vi "FPGA_main_Ctrl_v1.vi"() -> ()   [LabVIEW 2020]
doc: "Main FPGA VI\n- AI, Signal conditioning\n- AO, Feedback linearization\n- Controller"
uses:
  Components/FPGA TypeDefs/SelectDirection_Enum.ctl
  Components/FPGA TypeDefs/SelectExcitation_Enum.ctl
  Components/FPGA TypeDefs/SelectAOchannel_Enum.ctl
  Components/Controller/TypeDefs/2ndOrderTFnum.ctl
  Components/Controller/TypeDefs/2ndOrderTFden.ctl
  <vilib>/rvi/Emulation/niFpgaGetClockAttributes.vi
  <vilib>/rvi/Emulation/niFpgaSctlEmulationGetInTimedLoop.vi
  <vilib>/rvi/Emulation/niFpgaEmulationReportErrorSimple.vi
  <vilib>/rvi/eio/common/nirviEmuTemplateMethod_errors.vi
  <vilib>/rvi/Emulation/niFpgaEmulationIsFPGAContextNoSignature.vi
  <vilib>/rvi/errors/niFpgaSetErrorForExecOnDevCompSimple.vi
  <vilib>/rvi/eio/common/nirviEmuReportErrorAndStop.vi
  <vilib>/rvi/DataTransferAndStorage/Container/Common/niFpgaContainerGetUniqueNameForEmu.vi
  <vilib>/rvi/FIFO/Fifo_Resource/nirvififoEmulationSetSize.vi
  <vilib>/rvi/FIFO/Fifo_Resource/nirviFifoEmulationQueueMgr.vi
  <instcachedir>/0/nirviFifoEmulationQueueMgr_E5CAEC123FF24DC58D834DCA3CDAA9B5.lvgen/nirviFifoEmulationQueueMgr_E5CAEC123FF24DC58D834DCA3CDAA9B5_001.vi
  <vilib>/rvi/FIFO/Fifo_Resource/nirvififoEmulationDetermineInputValidOut.vi
  <vilib>/rvi/FIFO/Fifo_Resource/nirvififoEmulationCreateLock.vi
  <vilib>/rvi/Emulation/niFpgaProcessEmulError.vi
  <vilib>/rvi/FIFO/Fifo_Resource/nirvififoEmulationObtainLock.vi
  <vilib>/rvi/FIFO/Fifo_Resource/nirvififoEmulationReleaseLock.vi
  <vilib>/rvi/occurrence/nirviWaitOnOccurrenceBase.vi
  <vilib>/rvi/errors/nirviReportUnexpectedCaseInternalError.vi
  <vilib>/rvi/errors/nirviReportUnexpectedCaseInternalError (U32).vi
  <vilib>/rvi/Emulation/niFpgaCriticalErrorInLSC.vi
  <vilib>/Utility/error.llb/Clear Errors.vi
  Components/PositionMeas/MovingAverage/256ptMovingAvg.vi
  Components/PositionMeas/MovingAverage/64ptMovingAvg.vi
  <vilib>/rvi/DataTransferAndStorage/Container/Common/niFpgaContainerSetEmuInfo.vi
  <vilib>/eio/EIONode/EIONode.xnode
  <vilib>/rvi/DataTransferAndStorage/Container/XNode/niFpgaContainer.xnode
  <vilib>/rvi/FIFO/Fifo_Resource/nirvififoEmulationWrite.vi
  <vilib>/rvi/FIFO/Fifo_Resource/nirvififoEmulationRead.vi
  <vilib>/rvi/FXPMathLib/FxpSub/XNode/nifxpmath_Sub.xnode
  <vilib>/rvi/FXPMathLib/FxpAdd/XNode/nifxpmath_Add.xnode
  <vilib>/rvi/LocalResourceManager/LocalResourceManager.xnode
  Components/PositionMeas/MovingAverage/MovingAvg.lvlib
  Components/PositionMeas/PositionMeas.lvlib
  Components/Controller/Controller.lvlib
  <vilib>/rvi/FXPMathLib/sim/FxpSim.dll
  Components/ReferenceGen/ReferenceGen.lvlib
  Components/CtrlEff/CtrlEff.lvlib
  Components/CtrlEff/Force2Volt/Force2Volt.lvlib
panel:
  in  "Numerator (b0, b1, b2) 5":T1=[0.0, 0.0, 0.0]
  in  "Denominator (a1, a2) 5":T2=[0.0, 0.0]
  in  "Denominator (a1, a2) 4":T2=[0.0, 0.0]
  in  "Denominator (a1, a2) 3":T2=[0.0, 0.0]
  in  "Denominator (a1, a2) 2":T2=[0.0, 0.0]
  in  "Numerator (b0, b1, b2) 4":T1=[0.0, 0.0, 0.0]
  in  "Numerator (b0, b1, b2) 3":T1=[0.0, 0.0, 0.0]
  in  "Numerator (b0, b1, b2) 2":T1=[0.0, 0.0, 0.0]
  in  "Denominator (a1, a2)":T2=[0.0, 0.0] format="%#_12g"
  in  "Numerator (b0, b1, b2)":T1=[0.0, 0.0, 0.0]
  in  "Current Sense Zero":fxp<+/-,25,5>[](array[numeric])=[0.0, 0.0, 0.0, 0.0, 0.0, 0.0]
  out "Total Ctrl Eff":fxp<+/-,25,5>[](array[numeric])
  in  "PosMeas_ZeroOffset":fxp<+/-,25,5>[](array[numeric])=[0.0, 0.0, 0.0, 0.0, 0.0]
  in  "AO enable?":bool
  out "Total PosRef":fxp<+/-,25,5>[](array[numeric])
  in  "Enable \nPos. Ref. Gen?":bool
  in  "Select Ref. direction":T3
  in  "PR Frequency [periods/tick]":fxp<+,32,0>
  in  "PR Amplitude [V]":fxp<+/-,25,5>
  in  "PR Excitation mode":T4
  out "Ref Gen Loop Time [ticks]":u32
  in  "Enable \nCtrl Eff dist?":bool
  in  "Enable \nAO dist?":bool
  in  "Select CE direction":T3
  in  "CE Frequency [periods/tick]":fxp<+,32,0>
  in  "CE Amplitude [V]":fxp<+/-,25,5>
  in  "CE Excitation mode":T4
  out "AO":fxp<+/-,20,5>[](array[numeric])
  in  "Run Controller?":bool
  in  "Ki*Ts":fxp<+,17,0>[](array[numeric])=[0.0, 0.0, 0.0, 0.0, 0.0] caption="Kp"
  out "U_Z,ThX,ThY,B,Bd":fxp<+/-,25,5>[](array[numeric])
  in  "Kp":fxp<+,17,17>[](array[numeric])=[0.0, 0.0, 0.0, 0.0, 0.0]
  out "Ctrl Loop\ntime [ticks]":u32
  in  "Z,ThX,ThY,B,Bd Ref":fxp<+/-,25,5>[](array[numeric])=[0.0, 0.0, 0.0, 0.0, 0.0]
  out "AI_HS":fxp<+/-,25,5>[](array[numeric])
  out "AI_LS":fxp<+/-,25,5>[](array[numeric])
  out "Z,ThX,ThY,B,Bd Meas":fxp<+/-,25,5>[](array[numeric])
  in  "Select AO channel":T5
  out "AO Loop time [ticks]":u32
  in  "AO Frequency [periods/tick]":fxp<+,32,0>
  in  "AO Amplitude [V]":fxp<+/-,25,5>
  in  "AO Excitation mode":T4
  out "AI LS 2 Loop time [ticks]":u32
  out "FPGA AI LS 2 FIFO\nOverflow?":bool
  out "AI LS 2 filter Loop time [ticks]":u32
  out "Current Sense":fxp<+/-,25,5>[](array[numeric])
  out "AI LS filter Loop time [ticks]":u32
  out "AI LS Loop time [ticks]":u16
  out "FPGA AI LS FIFO\nOverflow?":bool
  out "AI HS filter Loop time [ticks]":u32
  out "FPGA AI HS FIFO\nOverflow?":bool
  out "AI HS Loop time [ticks]":u32
  # "1 tick = 25 ns"
  # "2nd Order TF params"
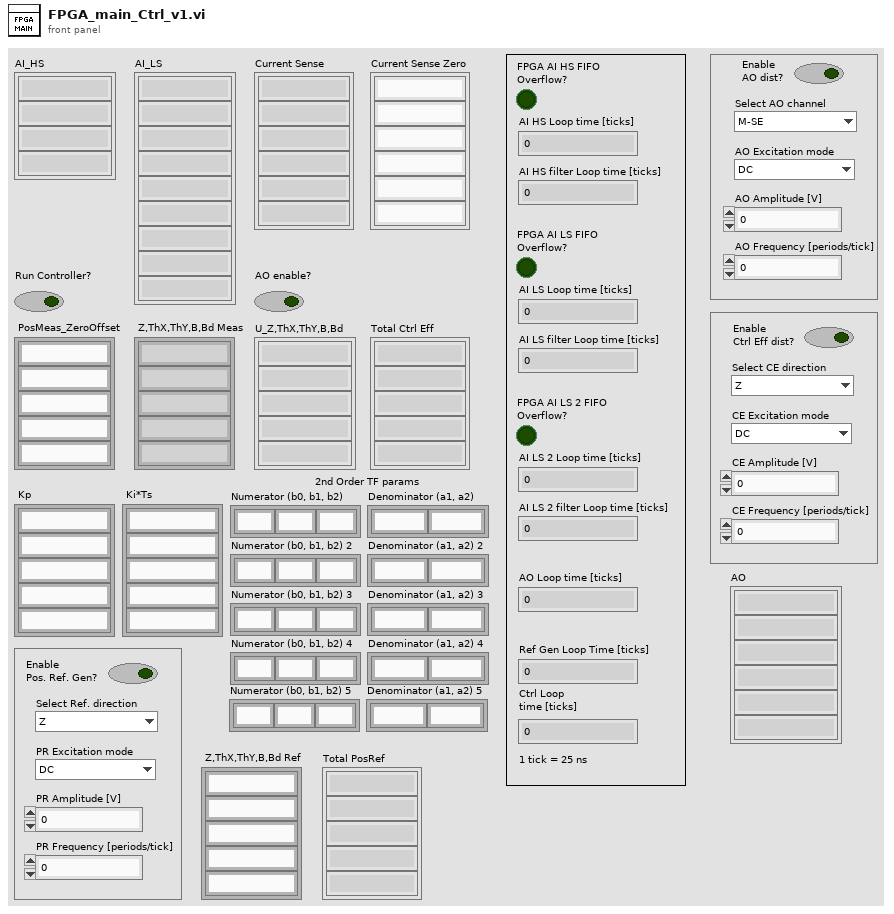
[diagram p1: front panel]
types:
  T1 = typedef "Controller.lvlib/2ndOrderTFnum.ctl" = fxp<+/-,28,2>[]
  T2 = typedef "Controller.lvlib/2ndOrderTFden.ctl" = fxp<+/-,28,2>[]
  T3 = typedef "SelectDirection_Enum.ctl" = enum8{"Z", "ThX", "ThY", "Bow", "B-d"}
  T4 = typedef "SelectExcitation_Enum.ctl" = enum8{"DC", "Sine", "Square", "WhiteNoise"}
  T5 = typedef "SelectAOchannel_Enum.ctl" = enum8{"M-SE", "M-NE", "M-NW", "M-SW", "M-CO", "M-CI"}
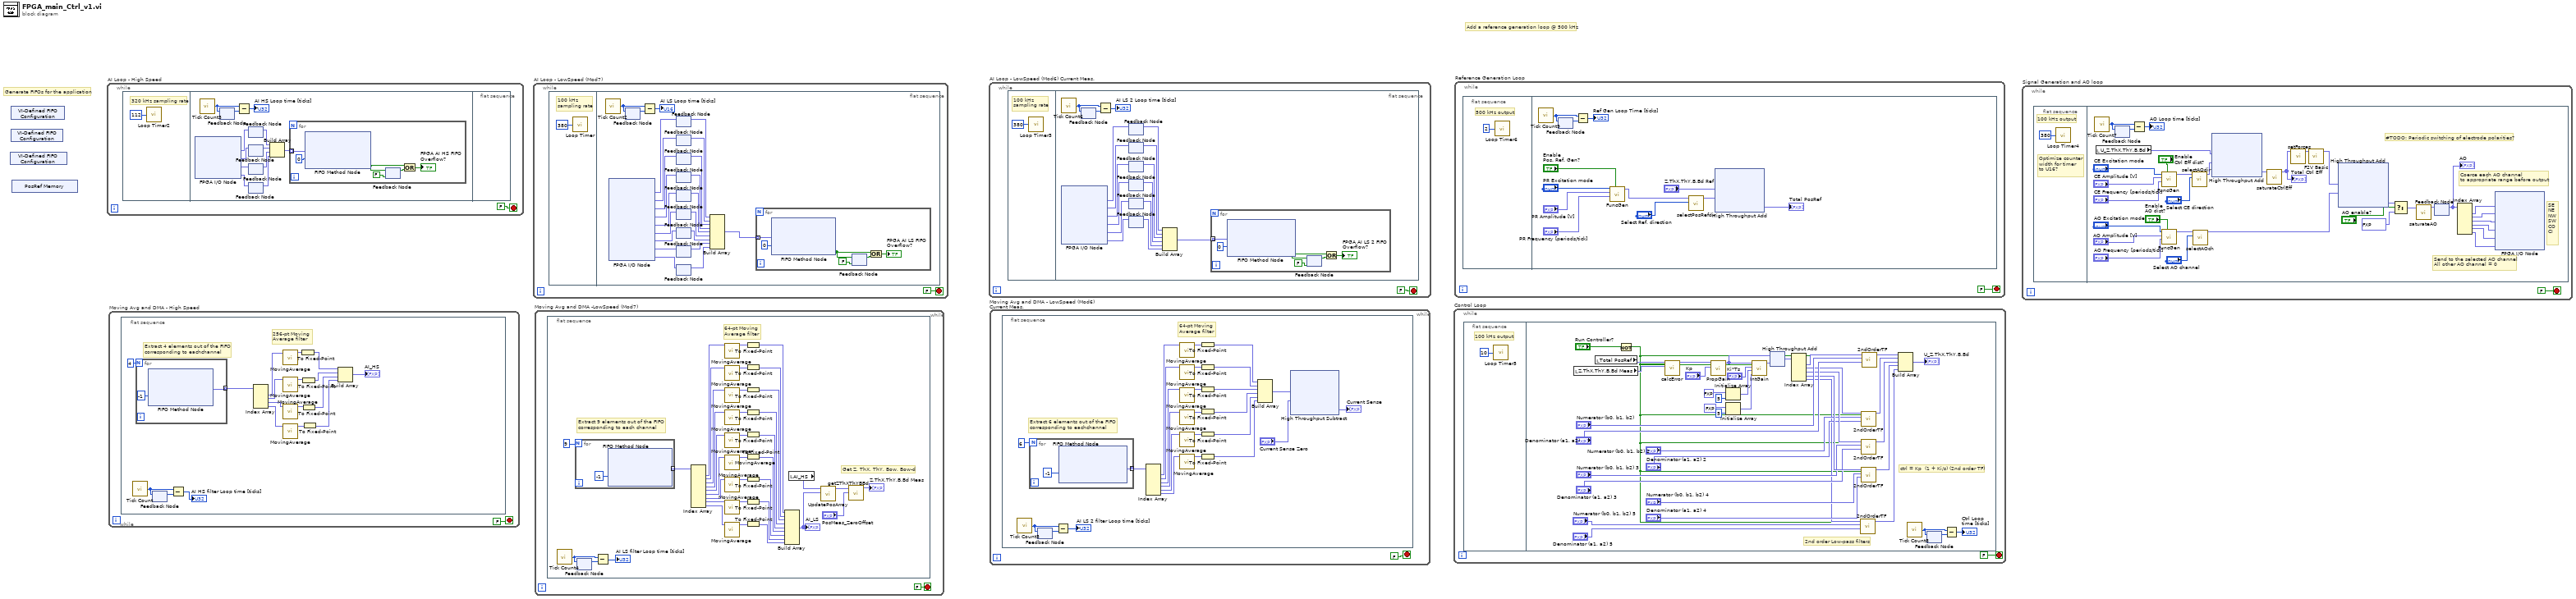
[diagram p0: block diagram]
diagram:
  # "Add a reference generation loop @ 500 kHz"
  # "Generate FIFOs for the application"
  n1 = xnode "VI-Defined FIFO Configuration"() -> ()  [unwired: 1 out]
  n2 = xnode "VI-Defined FIFO Configuration"() -> ()  [unwired: 1 out]
  n3 = xnode "VI-Defined FIFO Configuration"() -> ()  [unwired: 1 out]
  n4 = xnode "PosRef Memory"() -> ()  [unwired: 1 out]
  n5 = while "AI Loop - High Speed" {
    stop <- FALSE stop-if-true
    n6 = flat-sequence {
      frame #0 {
        # "320 kHz sampling rate"
        n7 = call "Loop Timer2"("Count(Ticks)"=u32 112) -> ()  [unwired: 1 out]
      }
      frame #1 {
        n8 = xnode "FPGA I/O Node"() -> ("Mod8/AI0"=w9:fxp<+/-,24,5>, "Mod8/AI1"=w8:fxp<+/-,24,5>, "Mod8/AI2"=w7:fxp<+/-,24,5>, "Mod8/AI3"=w6:fxp<+/-,24,5>)  [unwired: 4 in, 4 out]
        n9 = call "Tick Count3"() -> ("Tick Count(Ticks)"=w14:u32)
        n10 = feedback #1() -> (w13:u32)  [unwired: 1 in]
        n11 = feedback-in #1(w14) -> ()
        n12 = Subtract(x=w14, y=w13) -> (x-y=→"AI HS Loop time [ticks]":u32)
        n13 = feedback-in #2(w9) -> ()
        n14 = feedback #2() -> (w10:fxp<+/-,24,5>)  [unwired: 1 in]
        n15 = feedback #3() -> (w5:fxp<+/-,24,5>)  [unwired: 1 in]
        n16 = feedback-in #3(w8) -> ()
        n17 = feedback #4() -> (w4:fxp<+/-,24,5>)  [unwired: 1 in]
        n18 = feedback-in #4(w7) -> ()
        n19 = feedback #5() -> (w3:fxp<+/-,24,5>)  [unwired: 1 in]
        n20 = feedback-in #5(w6) -> ()
        n21 = Build Array(w10, w5, w4, w3) -> (w11:fxp<+/-,24,5>[])
        n22 = for {
          tunnel: w11 -> [w19] mode=indexing
          n23 = xnode ("FIFO Method Node")("Element"=w19, "Timeout"=0) -> ("Timed Out?"=w16:bool)  [unwired: 1 in, 1 out]
          n24 = feedback-in #6(w16) -> ()
          n25 = feedback #6(FALSE ("Timed Out?")) -> (w17:bool)
          n26 = Or(x=w16, y=w17) -> (x .or. y?=→"FPGA AI HS FIFO\nOverflow?":bool)
        }
      }
      frame #2 {
      }
    }
  }
  n27 = while "Moving Avg and DMA - High Speed" {
    stop <- FALSE stop-if-true
    n28 = flat-sequence {
      frame #0 {
        # "256-pt Moving \nAverage filter"
        # "Extract 4 elements out of the FIFO \ncorresponding to eachchannel"
        n29 = call "Tick Count"() -> ("Tick Count(Ticks)"=w38:u32)
        n30 = for {
          N: 4 -> [_]
          tunnel: [w40] -> w35 mode=indexing
          n31 = xnode ("FIFO Method Node")("Timeout"=-1) -> ("Element"=w40:fxp<+/-,24,5>)  [unwired: 1 in, 2 out]
        }
        n32 = feedback #7() -> (w37:u32)  [unwired: 1 in]
        n33 = feedback-in #7(w38) -> ()
        n34 = Subtract(x=w38, y=w37) -> (x-y=→"AI HS filter Loop time [ticks]":u32)
        n35 = Index Array(array=w35) -> (element #1=w34:fxp<+/-,24,5>, element #2=w33:fxp<+/-,24,5>, element #3=w31:fxp<+/-,24,5>, element #4=w32:fxp<+/-,24,5>)  [unwired: 4 in]
        n36 = call-poly "MovingAverage.vi"("Raw input"=w34) -> ("Output"=w30:fxp<+/-,28,5>)  [unwired: 10 in]
        n37 = call-poly "MovingAverage.vi"("Raw input"=w33) -> ("Output"=w29:fxp<+/-,28,5>)  [unwired: 10 in]
        n38 = call-poly "MovingAverage.vi"("Raw input"=w31) -> ("Output"=w28:fxp<+/-,28,5>)  [unwired: 10 in]
        n39 = call-poly "MovingAverage.vi"("Raw input"=w32) -> ("Output"=w27:fxp<+/-,28,5>)  [unwired: 10 in]
        n40 = To Fixed-Point(number=w30) -> (fixed-point=w26:fxp<+/-,25,5>)  [unwired: 1 in]
        n41 = To Fixed-Point(number=w29) -> (fixed-point=w25:fxp<+/-,25,5>)  [unwired: 1 in]
        n42 = To Fixed-Point(number=w28) -> (fixed-point=w24:fxp<+/-,25,5>)  [unwired: 1 in]
        n43 = To Fixed-Point(number=w27) -> (fixed-point=w23:fxp<+/-,25,5>)  [unwired: 1 in]
        n44 = Build Array(w26, w25, w24, w23) -> (→"AI_HS":fxp<+/-,25,5>[])
      }
    }
  }
  n45 = while "AI Loop - LowSpeed (Mod7)" {
    stop <- FALSE stop-if-true
    n46 = flat-sequence {
      frame #0 {
        # "100 kHz \nsampling rate"
        n47 = call "Loop Timer"("Count(Ticks)"=u16 380) -> ()  [unwired: 1 out]
      }
      frame #1 {
        n48 = call "Tick Count2"() -> ("Tick Count(Ticks)"=w65:u16)
        n49 = xnode "FPGA I/O Node"() -> ("Mod7/AI0"=w61:fxp<+/-,24,5>, "Mod7/AI1"=w60:fxp<+/-,24,5>, "Mod7/AI2"=w59:fxp<+/-,24,5>, "Mod7/AI3"=w58:fxp<+/-,24,5>, "Mod7/AI4"=w57:fxp<+/-,24,5>, "Mod7/AI5"=w56:fxp<+/-,24,5>, "Mod7/AI6"=w55:fxp<+/-,24,5>, "Mod7/AI7"=w54:fxp<+/-,24,5>, "Mod7/AI8"=w53:fxp<+/-,24,5>)  [unwired: 9 in, 9 out]
        n50 = feedback #8() -> (w64:u16)  [unwired: 1 in]
        n51 = feedback-in #8(w65) -> ()
        n52 = Subtract(x=w65, y=w64) -> (x-y=→"AI LS Loop time [ticks]":u16)
        n53 = feedback #9() -> (w52:fxp<+/-,24,5>)  [unwired: 1 in]
        n54 = feedback-in #9(w61) -> ()
        n55 = feedback #10() -> (w51:fxp<+/-,24,5>)  [unwired: 1 in]
        n56 = feedback-in #10(w60) -> ()
        n57 = feedback #11() -> (w50:fxp<+/-,24,5>)  [unwired: 1 in]
        n58 = feedback-in #11(w59) -> ()
        n59 = feedback #12() -> (w49:fxp<+/-,24,5>)  [unwired: 1 in]
        n60 = feedback-in #12(w58) -> ()
        n61 = feedback #13() -> (w48:fxp<+/-,24,5>)  [unwired: 1 in]
        n62 = feedback-in #13(w57) -> ()
        n63 = feedback #14() -> (w47:fxp<+/-,24,5>)  [unwired: 1 in]
        n64 = feedback-in #14(w56) -> ()
        n65 = feedback #15() -> (w46:fxp<+/-,24,5>)  [unwired: 1 in]
        n66 = feedback-in #15(w55) -> ()
        n67 = feedback #16() -> (w45:fxp<+/-,24,5>)  [unwired: 1 in]
        n68 = feedback-in #16(w54) -> ()
        n69 = feedback #17() -> (w44:fxp<+/-,24,5>)  [unwired: 1 in]
        n70 = feedback-in #17(w53) -> ()
        n71 = Build Array(w52, w51, w50, w49, w48, w47, w46, w45, w44) -> (w62:fxp<+/-,24,5>[])
        n72 = for {
          tunnel: w62 -> [w66] mode=indexing
          n73 = xnode ("FIFO Method Node")("Element"=w66, "Timeout"=0) -> ("Timed Out?"=w68:bool)  [unwired: 1 in, 1 out]
          n74 = feedback-in #18(w68) -> ()
          n75 = feedback #18(FALSE ("Timed Out?")) -> (w69:bool)
          n76 = Or(x=w68, y=w69) -> (x .or. y?=→"FPGA AI LS FIFO\nOverflow?":bool)
        }
      }
    }
  }
  n77 = while "Moving Avg and DMA -LowSpeed (Mod7)" {
    stop <- FALSE stop-if-true
    n78 = flat-sequence {
      frame #0 {
        # "Get Z, ThX, ThY, Bow, Bow-d"
        # "64-pt Moving \nAverage filter"
        # "Extract 9 elements out of the FIFO \ncorresponding to each channel"
        n79 = call "Tick Count4"() -> ("Tick Count(Ticks)"=w108:u32)
        n80 = for {
          N: 9 -> [_]
          tunnel: [w110] -> w105 mode=indexing
          n81 = xnode ("FIFO Method Node")("Timeout"=-1) -> ("Element"=w110:fxp<+/-,24,5>)  [unwired: 1 in, 2 out]
        }
        n82 = feedback #19() -> (w107:u32)  [unwired: 1 in]
        n83 = feedback-in #19(w108) -> ()
        n84 = Subtract(x=w108, y=w107) -> (x-y=→"AI LS filter Loop time [ticks]":u32)
        n85 = Index Array(array=w105) -> (element #1=w104:fxp<+/-,24,5>, element #2=w103:fxp<+/-,24,5>, element #3=w102:fxp<+/-,24,5>, element #4=w101:fxp<+/-,24,5>, element #5=w100:fxp<+/-,24,5>, element #6=w99:fxp<+/-,24,5>, element #7=w98:fxp<+/-,24,5>, element #8=w97:fxp<+/-,24,5>, element #9=w96:fxp<+/-,24,5>)  [unwired: 9 in]
        n86 = call-poly "MovingAverage.vi"("Raw input"=w104) -> ("Output"=w95:fxp<+/-,28,5>)  [unwired: 10 in]
        n87 = call-poly "MovingAverage.vi"("Raw input"=w103) -> ("Output"=w94:fxp<+/-,28,5>)  [unwired: 10 in]
        n88 = call-poly "MovingAverage.vi"("Raw input"=w102) -> ("Output"=w93:fxp<+/-,28,5>)  [unwired: 10 in]
        n89 = call-poly "MovingAverage.vi"("Raw input"=w101) -> ("Output"=w92:fxp<+/-,28,5>)  [unwired: 10 in]
        n90 = call-poly "MovingAverage.vi"("Raw input"=w100) -> ("Output"=w91:fxp<+/-,28,5>)  [unwired: 10 in]
        n91 = call-poly "MovingAverage.vi"("Raw input"=w99) -> ("Output"=w90:fxp<+/-,28,5>)  [unwired: 10 in]
        n92 = call-poly "MovingAverage.vi"("Raw input"=w98) -> ("Output"=w89:fxp<+/-,28,5>)  [unwired: 10 in]
        n93 = call-poly "MovingAverage.vi"("Raw input"=w97) -> ("Output"=w88:fxp<+/-,28,5>)  [unwired: 10 in]
        n94 = call-poly "MovingAverage.vi"("Raw input"=w96) -> ("Output"=w87:fxp<+/-,28,5>)  [unwired: 10 in]
        n95 = To Fixed-Point(number=w95) -> (fixed-point=w86:fxp<+/-,25,5>)  [unwired: 1 in]
        n96 = To Fixed-Point(number=w94) -> (fixed-point=w85:fxp<+/-,25,5>)  [unwired: 1 in]
        n97 = To Fixed-Point(number=w93) -> (fixed-point=w84:fxp<+/-,25,5>)  [unwired: 1 in]
        n98 = To Fixed-Point(number=w92) -> (fixed-point=w83:fxp<+/-,25,5>)  [unwired: 1 in]
        n99 = To Fixed-Point(number=w91) -> (fixed-point=w82:fxp<+/-,25,5>)  [unwired: 1 in]
        n100 = To Fixed-Point(number=w90) -> (fixed-point=w81:fxp<+/-,25,5>)  [unwired: 1 in]
        n101 = To Fixed-Point(number=w89) -> (fixed-point=w80:fxp<+/-,25,5>)  [unwired: 1 in]
        n102 = To Fixed-Point(number=w88) -> (fixed-point=w79:fxp<+/-,25,5>)  [unwired: 1 in]
        n103 = To Fixed-Point(number=w87) -> (fixed-point=w78:fxp<+/-,25,5>)  [unwired: 1 in]
        n104 = Build Array(w86, w85, w84, w83, w82, w81, w80, w79, w78) -> (w76:fxp<+/-,25,5>[])
        "AI_LS" <- w76
        n105 = local read "AI_HS"() -> (w77:fxp<+/-,25,5>[])
        n106 = call "UpdatePosArray.vi"("AI_LS"=w76, "AI_HS"=w77) -> ("AI_HS_LS"=w75:fxp<+/-,25,5>[])  [unwired: 9 in]
        n107 = call "getZThXThYBBd.vi"("PosMeas_ZeroOffset"="PosMeas_ZeroOffset", "PosMeas_Array In"=w75) -> ("Z,ThX,ThY,B,Bd_out"=→"Z,ThX,ThY,B,Bd Meas":fxp<+/-,25,5>[])  [unwired: 9 in]
      }
    }
  }
  n108 = while "AI Loop - LowSpeed (Mod6) Current Meas." {
    stop <- FALSE stop-if-true
    n109 = flat-sequence {
      frame #0 {
        # "100 kHz \nsampling rate"
        n110 = call "Loop Timer3"("Count(Ticks)"=u32 380) -> ()  [unwired: 1 out]
      }
      frame #1 {
        n111 = call "Tick Count6"() -> ("Tick Count(Ticks)"=w129:u32)
        n112 = xnode "FPGA I/O Node"() -> ("Mod6/AI0"=w125:fxp<+/-,24,5>, "Mod6/AI1"=w118:fxp<+/-,24,5>, "Mod6/AI2"=w117:fxp<+/-,24,5>, "Mod6/AI3"=w116:fxp<+/-,24,5>, "Mod6/AI4"=w115:fxp<+/-,24,5>, "Mod6/AI5"=w114:fxp<+/-,24,5>)  [unwired: 6 in, 6 out]
        n113 = feedback #20() -> (w128:u32)  [unwired: 1 in]
        n114 = feedback-in #20(w129) -> ()
        n115 = Subtract(x=w129, y=w128) -> (x-y=→"AI LS 2 Loop time [ticks]":u32)
        n116 = feedback #21() -> (w124:fxp<+/-,24,5>)  [unwired: 1 in]
        n117 = feedback-in #21(w125) -> ()
        n118 = feedback #22() -> (w123:fxp<+/-,24,5>)  [unwired: 1 in]
        n119 = feedback-in #22(w118) -> ()
        n120 = feedback #23() -> (w122:fxp<+/-,24,5>)  [unwired: 1 in]
        n121 = feedback-in #23(w117) -> ()
        n122 = feedback #24() -> (w121:fxp<+/-,24,5>)  [unwired: 1 in]
        n123 = feedback-in #24(w116) -> ()
        n124 = feedback #25() -> (w120:fxp<+/-,24,5>)  [unwired: 1 in]
        n125 = feedback-in #25(w115) -> ()
        n126 = feedback #26() -> (w119:fxp<+/-,24,5>)  [unwired: 1 in]
        n127 = feedback-in #26(w114) -> ()
        n128 = Build Array(w124, w123, w122, w121, w120, w119) -> (w126:fxp<+/-,24,5>[])
        n129 = for {
          tunnel: w126 -> [w130] mode=indexing
          n130 = xnode ("FIFO Method Node")("Element"=w130, "Timeout"=0) -> ("Timed Out?"=w132:bool)  [unwired: 1 in, 1 out]
          n131 = feedback-in #27(w132) -> ()
          n132 = feedback #27(FALSE ("Timed Out?")) -> (w133:bool)
          n133 = Or(x=w132, y=w133) -> (x .or. y?=→"FPGA AI LS 2 FIFO\nOverflow?":bool)
        }
      }
    }
  }
  n134 = while "Moving Avg and DMA - LowSpeed (Mod6) Current Meas." {
    stop <- FALSE stop-if-true
    n135 = flat-sequence {
      frame #0 {
        # "64-pt Moving \nAverage filter"
        # "Extract 6 elements out of the FIFO \ncorresponding to eachchannel"
        n136 = call "Tick Count5"() -> ("Tick Count(Ticks)"=w161:u32)
        n137 = for {
          N: 6 -> [_]
          tunnel: [w163] -> w158 mode=indexing
          n138 = xnode ("FIFO Method Node")("Timeout"=-1) -> ("Element"=w163:fxp<+/-,24,5>)  [unwired: 1 in, 2 out]
        }
        n139 = feedback #28() -> (w160:u32)  [unwired: 1 in]
        n140 = feedback-in #28(w161) -> ()
        n141 = Subtract(x=w161, y=w160) -> (x-y=→"AI LS 2 filter Loop time [ticks]":u32)
        n142 = Index Array(array=w158) -> (element #1=w156:fxp<+/-,24,5>, element #2=w155:fxp<+/-,24,5>, element #3=w154:fxp<+/-,24,5>, element #4=w153:fxp<+/-,24,5>, element #5=w152:fxp<+/-,24,5>, element #6=w151:fxp<+/-,24,5>)  [unwired: 6 in]
        n143 = call-poly "MovingAverage.vi"("Raw input"=w156) -> ("Output"=w150:fxp<+/-,28,5>)  [unwired: 10 in]
        n144 = call-poly "MovingAverage.vi"("Raw input"=w155) -> ("Output"=w149:fxp<+/-,28,5>)  [unwired: 10 in]
        n145 = call-poly "MovingAverage.vi"("Raw input"=w154) -> ("Output"=w148:fxp<+/-,28,5>)  [unwired: 10 in]
        n146 = call-poly "MovingAverage.vi"("Raw input"=w153) -> ("Output"=w147:fxp<+/-,28,5>)  [unwired: 10 in]
        n147 = call-poly "MovingAverage.vi"("Raw input"=w152) -> ("Output"=w146:fxp<+/-,28,5>)  [unwired: 10 in]
        n148 = call-poly "MovingAverage.vi"("Raw input"=w151) -> ("Output"=w145:fxp<+/-,28,5>)  [unwired: 10 in]
        n149 = To Fixed-Point(number=w150) -> (fixed-point=w157:fxp<+/-,25,5>)  [unwired: 1 in]
        n150 = To Fixed-Point(number=w149) -> (fixed-point=w144:fxp<+/-,25,5>)  [unwired: 1 in]
        n151 = To Fixed-Point(number=w148) -> (fixed-point=w143:fxp<+/-,25,5>)  [unwired: 1 in]
        n152 = To Fixed-Point(number=w147) -> (fixed-point=w142:fxp<+/-,25,5>)  [unwired: 1 in]
        n153 = To Fixed-Point(number=w146) -> (fixed-point=w141:fxp<+/-,25,5>)  [unwired: 1 in]
        n154 = To Fixed-Point(number=w145) -> (fixed-point=w140:fxp<+/-,25,5>)  [unwired: 1 in]
        n155 = Build Array(w157, w144, w143, w142, w141, w140) -> (w139:fxp<+/-,25,5>[])
        n156 = xnode "High Throughput Subtract"("x"=w139, "y"="Current Sense Zero") -> ("x-y"=→"Current Sense":fxp<+/-,25,5>[])
      }
    }
  }
  n157 = while "Control Loop" {
    stop <- FALSE stop-if-true
    n158 = flat-sequence {
      frame #0 {
        # "100 kHz output"
        n159 = call "Loop Timer5"("Count(uSec)"=u8 10 ("Count(Ticks)")) -> ()  [unwired: 1 out]
      }
      frame #1 {
        # "ctrl = Kp  (1 + Ki/s) (2nd order TF)"
        # "2nd order Low-pass filters"
        n160 = local read "Z,ThX,ThY,B,Bd Meas"() -> (w201:fxp<+/-,25,5>[])
        n161 = local read "Total PosRef"() -> (w200:fxp<+/-,25,5>[])
        n162 = Not(x="Run Controller?") -> (.not. x?=w167:bool)
        n163 = call "calcError.vi"("Initialize?"=w167, "Z,ThX,ThY,Bow Meas"=w201, "Z,ThX,ThY,Bow Ref"=w200) -> ("Z,ThX,ThY,Bow Error"=w206:fxp<+/-,25,5>[])  [unwired: 8 in]
        n164 = call "PropGain.vi"("Initialize?"=w167, "Kp"="Kp", "Ctrl Effort In"=w206) -> ("Ctrl Effort Out"=w203:fxp<+/-,25,5>[])  [unwired: 8 in]
        n165 = Initialize Array(fxp<+/-,25,5> 10.0, 5 ("dimension size")) -> (w180:fxp<+/-,25,5>[])
        n166 = Initialize Array(fxp<+/-,25,5> -10.0, 5 ("dimension size")) -> (w175:fxp<+/-,25,5>[])
        n167 = call "IntGain.vi"("Initialize?"=w167, "Lower Limit (-10)"=w175, "Upper Limit (10)"=w180, "Ki*Ts"="Ki*Ts", "Ctrl Effort In"=w203) -> ("Ctrl Effort Out"=w202:fxp<+/-,25,5>[])  [unwired: 6 in]
        n168 = xnode ("High Throughput Add")("x"=w203, "y"=w202) -> ("x+y"=w198:fxp<+/-,25,5>[])
        n169 = Index Array(array=w198) -> (element #1=w197:fxp<+/-,25,5>, element #2=w194:fxp<+/-,25,5>, element #3=w193:fxp<+/-,25,5>, element #4=w192:fxp<+/-,25,5>, element #5=w169:fxp<+/-,25,5>)  [unwired: 5 in]
        n170 = call "2ndOrderTF.vi"("Initialize?"=w167, "Denominator (a1, a2)"="Denominator (a1, a2) 5", "Numerator (b0, b1, b2)"="Numerator (b0, b1, b2) 5", "Ctrl Effort In"=w169) -> ("Ctrl Effort Out"=w168:fxp<+/-,25,5>)  [unwired: 7 in]
        n171 = call "2ndOrderTF.vi"("Initialize?"=w167, "Denominator (a1, a2)"="Denominator (a1, a2) 2", "Numerator (b0, b1, b2)"="Numerator (b0, b1, b2) 2", "Ctrl Effort In"=w194) -> ("Ctrl Effort Out"=w184:fxp<+/-,25,5>)  [unwired: 7 in]
        n172 = call "2ndOrderTF.vi"("Initialize?"=w167, "Denominator (a1, a2)"="Denominator (a1, a2) 3", "Numerator (b0, b1, b2)"="Numerator (b0, b1, b2) 3", "Ctrl Effort In"=w193) -> ("Ctrl Effort Out"=w183:fxp<+/-,25,5>)  [unwired: 7 in]
        n173 = call "2ndOrderTF.vi"("Initialize?"=w167, "Denominator (a1, a2)"="Denominator (a1, a2) 4", "Numerator (b0, b1, b2)"="Numerator (b0, b1, b2) 4", "Ctrl Effort In"=w192) -> ("Ctrl Effort Out"=w182:fxp<+/-,25,5>)  [unwired: 7 in]
        n174 = call "2ndOrderTF.vi"("Initialize?"=w167, "Denominator (a1, a2)"="Denominator (a1, a2)", "Numerator (b0, b1, b2)"="Numerator (b0, b1, b2)", "Ctrl Effort In"=w197) -> ("Ctrl Effort Out"=w185:fxp<+/-,25,5>)  [unwired: 7 in]
        n175 = Build Array(w185, w184, w183, w182, w168) -> (→"U_Z,ThX,ThY,B,Bd":fxp<+/-,25,5>[])
        n176 = call "Tick Count8"() -> ("Tick Count(Ticks)"=w174:u32)
        n177 = feedback #29() -> (w173:u32)  [unwired: 1 in]
        n178 = feedback-in #29(w174) -> ()
        n179 = Subtract(x=w174, y=w173) -> (x-y=→"Ctrl Loop\ntime [ticks]":u32)
      }
    }
  }
  n180 = while "Reference Generation Loop" {
    stop <- FALSE stop-if-true
    n181 = flat-sequence {
      frame #0 {
        # "500 kHz output"
        n182 = call "Loop Timer6"("Count(uSec)"=u8 2 ("Count(Ticks)")) -> ()  [unwired: 1 out]
      }
      frame #1 {
        n183 = call "Tick Count9"() -> ("Tick Count(Ticks)"=w218:u32)
        n184 = feedback #30() -> (w219:u32)  [unwired: 1 in]
        n185 = feedback-in #30(w218) -> ()
        n186 = Subtract(x=w218, y=w219) -> (x-y=→"Ref Gen Loop Time [ticks]":u32)
        n187 = call "FuncGen.vi"("Enable?"="Enable \nPos. Ref. Gen?", "Frequency [periods/tick]"="PR Frequency [periods/tick]", "Amplitude [V]"="PR Amplitude [V]", "Excitation mode"="PR Excitation mode") -> ("Output [V]"=w212:fxp<+/-,25,5>)  [unwired: 7 in]
        n188 = call "selectPosRefdir.vi"("Select direction"="Select Ref. direction", "signal input"=w212) -> ("Ctrl Eff Array Out"=w211:fxp<+/-,25,5>[])  [unwired: 9 in]
        n189 = xnode ("High Throughput Add")("x"="Z,ThX,ThY,B,Bd Ref", "y"=w211) -> ("x+y"=→"Total PosRef":fxp<+/-,25,5>[])
      }
    }
  }
  n190 = while "Signal Generation and AO loop" {
    stop <- FALSE stop-if-true
    n191 = flat-sequence {
      frame #0 {
        # "Optimize counter\nwidth for timer \nto U16?"
        # "100 kHz output"
        n192 = call "Loop Timer4"("Count(Ticks)"=u32 380) -> ()  [unwired: 1 out]
      }
      frame #1 {
        # "#TODO: Periodic switching of electrode polarities?"
        # "Coerce each AO channel\nto appropriate range before output"
        # "SE\nNE\nNW\nSW\nCO\nCI"
        # "Send to the selected AO channel\nAll other AO channel = 0"
        n193 = call "Tick Count7"() -> ("Tick Count(Ticks)"=w256:u32)
        n194 = local read "U_Z,ThX,ThY,B,Bd"() -> (w228:fxp<+/-,25,5>[])
        n195 = feedback #31() -> (w255:u32)  [unwired: 1 in]
        n196 = feedback-in #31(w256) -> ()
        n197 = Subtract(x=w256, y=w255) -> (x-y=→"AO Loop time [ticks]":u32)
        n198 = call "FuncGen.vi"("Enable?"="Enable \nCtrl Eff dist?", "Frequency [periods/tick]"="CE Frequency [periods/tick]", "Amplitude [V]"="CE Amplitude [V]", "Excitation mode"="CE Excitation mode") -> ("Output [V]"=w235:fxp<+/-,25,5>)  [unwired: 7 in]
        n199 = call "FuncGen.vi"("Enable?"="Enable \nAO dist?", "Frequency [periods/tick]"="AO Frequency [periods/tick]", "Amplitude [V]"="AO Amplitude [V]", "Excitation mode"="AO Excitation mode") -> ("Output [V]"=w244:fxp<+/-,25,5>)  [unwired: 7 in]
        n200 = call "selectAOdir.vi"("Select direction"="Select CE direction", "signal input"=w235) -> ("Ctrl Eff Array Out"=w227:fxp<+/-,25,5>[])  [unwired: 9 in]
        n201 = call "selectAOch.vi"("Select AO channel"="Select AO channel", "signal input"=w244) -> ("AO Array Out"=w242:fxp<+/-,20,5>[])  [unwired: 9 in]
        n202 = xnode ("High Throughput Add")("x"=w228, "y"=w227) -> ("x+y"=w226:fxp<+/-,25,5>[])
        n203 = call "saturateCtrlEff.vi"("Array In"=w226) -> ("Array Out"=w223:fxp<+/-,25,5>[])  [unwired: 10 in]
        "Total Ctrl Eff" <- w223
        n204 = call "setForces.vi"("CtrlEffArray In"=w223) -> ("ForceArray Out"=w240:fxp<+/-,25,5>[])  [unwired: 10 in]
        n205 = call "F2V Basic.vi"("ForceArray In"=w240) -> ("ElectrodeVoltageArray Out"=w239:fxp<+/-,20,5>[])  [unwired: 10 in]
        n206 = xnode ("High Throughput Add")("x"=w239, "y"=w242) -> ("x+y"=w233:fxp<+/-,20,5>[])
        n207 = Select(t=w233, s="AO enable?", f=fxp<+/-,20,5>[] [0.0, 0.0, 0.0, 0.0, 0.0, 0.0]) -> (s? t:f=w225:fxp<+/-,20,5>[])
        n208 = call "saturateAO.vi"("Array In"=w225) -> ("Array Out"=w224:fxp<+/-,20,5>[])  [unwired: 10 in]
        n209 = feedback-in #32(w224) -> ()
        n210 = feedback #32() -> (w241:fxp<+/-,20,5>[])  [unwired: 1 in]
        "AO" <- w241
        n211 = Index Array(array=w241) -> (element #1=w253:fxp<+/-,20,5>, element #2=w252:fxp<+/-,20,5>, element #3=w251:fxp<+/-,20,5>, element #4=w250:fxp<+/-,20,5>, element #5=w249:fxp<+/-,20,5>, element #6=w248:fxp<+/-,20,5>)  [unwired: 6 in]
        n212 = xnode "FPGA I/O Node"("Mod3/AO0"=w253, "Mod3/AO1"=w252, "Mod3/AO2"=w251, "Mod3/AO3"=w250, "Mod4/AO0"=w249, "Mod4/AO1"=w248) -> ()  [unwired: 6 in, 6 out]
      }
    }
  }
